vi "NewMessageToSend.vi"(6 "MessageType":T1, 8 "error in (no error)":errorcluster, 9 "Connection Number":i32, 10 "Message":string, 11 "TCP_ClientWindow_Controller in":refnum<class "TCP_ClientWindow_Controller.lvclass">) -> (0 "error out":errorcluster, 3 "TCP_ClientWindow_Controller out":refnum<class "TCP_ClientWindow_Controller.lvclass">)   [LabVIEW 2023, in "TCP_Client_Window.lvlib" / "TCP_ClientWindow_Controller.lvclass"]
uses:
  TCP_ClientWindow_Controller.lvclass
  TCP_Server_Connection_Handler/TypeDefinitions/messageType.ctl
  TCP_Server_Connection_Handler/TCP_Server_Connection_Handler.lvlib
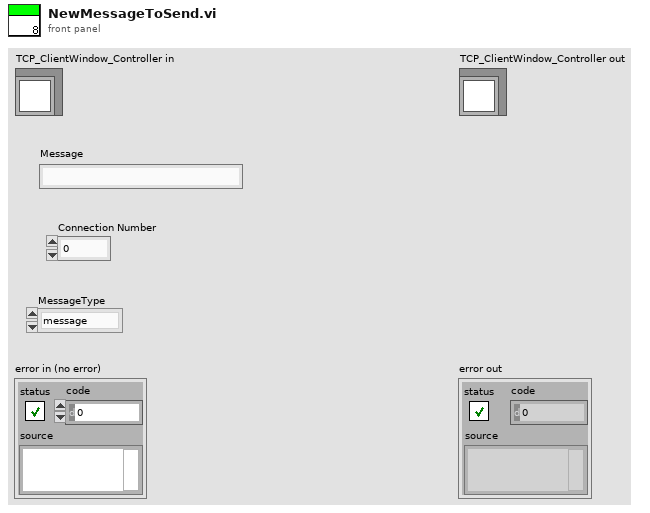
[diagram p1: front panel]
types:
  T1 = typedef "TCP_Server_Connection_Handler.lvlib/messageType.ctl" = enum16{"message", "file", "get", "ShutDown"}
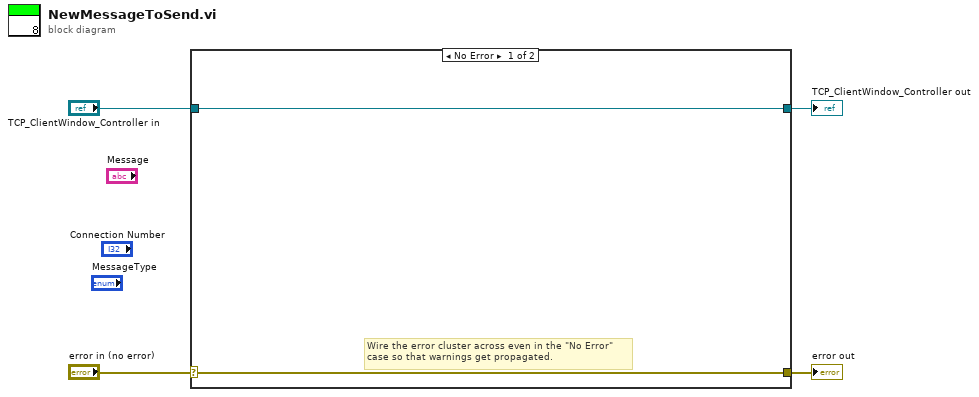
[diagram p0: block diagram]
diagram:
  n1 = case shown="No Error" "error in (no error)" {
    selector: "error in (no error)" -> [w5 w8]
    tunnel: [w5 w8] -> w3
    tunnel: [w6 w7] -> w1
    tunnel: "TCP_ClientWindow_Controller in" -> [w6 w7]
    frame No Error {
      # "Wire the error cluster across even in the \"No Error\"\ncase so that warnings get propagated."
    }
    frame Error {
    }
  }
  "error out" <- w3
  "TCP_ClientWindow_Controller out" <- w1
